vi "Binary to Nomal.vi"(0 "Module Type":T1=enum."NI 9215", 5 "Channel Calibration":cluster{"LSB Weight":u32, "Offset":i32}, 9 "Numeric":i32) -> (4 "Units":enum8{"mA", "V", "V/V", "Ohms"}(ring), 10 "data":dbl)   [LabVIEW 2018]
doc: "Converts a binary value to its nominal value equivalent.."
uses:
  <vilib>/LabVIEW Targets/FPGA/cRIO/shared/nicrio_ModuleControls/nicrio_calibrationModTypeEnum.ctl
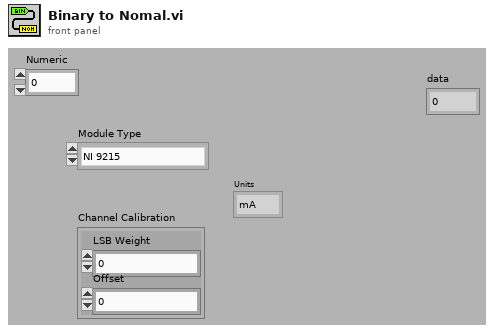
[diagram p1: front panel]
types:
  T1 = typedef "nicrio_calibrationModTypeEnum.ctl" = enum8{"NI 9201", "NI 9203 (4-20 mA range)", "NI 9203 (+/- 20 mA range)", "NI 9205", "NI 9206", "NI 9215", "NI 9221", "NI 9229", "NI 9233", "NI 9234", "NI 9237", "NI 9239", "NI 9263", "NI 9264", "NI 9265", "NI 9217", "NI 9236", "NI 9235", "NI 9225", "NI 9227", "NI 9269", "NI 9222", "NI 9223", "NI 9232", "NI 9381 (AI)", "NI 9381 (AO)", "NI 9220", "NI 9238", "NI 9218 (+/- 60 V range)", "NI 9218 (+/- 16 V range)", "NI 9218 (+/- 65 mV range)", "NI 9218 (+/- 5V IEPE range)", "NI 9218 (+/- 20 mA range)", "NI 9218 (+/- 22 mV/V range)", "NI 9260", "NI 9216", "NI 9226", "NI 9246", "NI 9247", "NI 9230", "NI 9266", "Ni 9775  (AI)", "NI 9775 (Trigger Level)", "NI 9775 (Hysteresis Level)", "NI 9684 (+/- 10 V range)", "NI 9684 (+/- 5 V range)"}
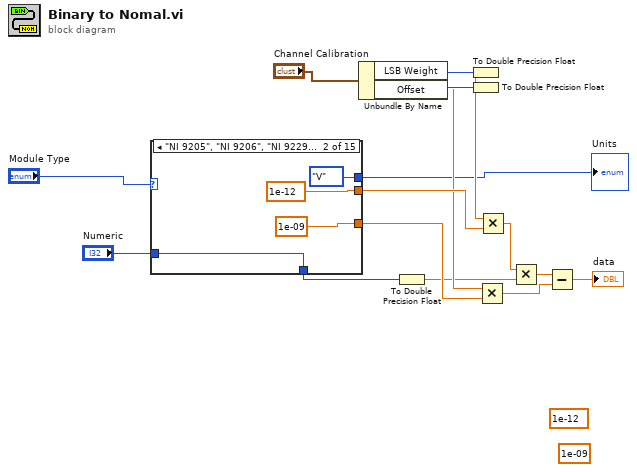
[diagram p0: block diagram]
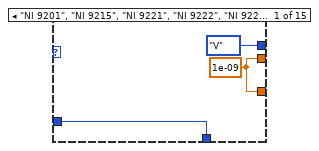
[diagram p2: hidden frame]
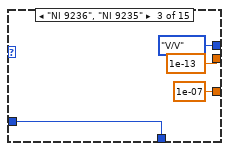
[diagram p3: hidden frame]
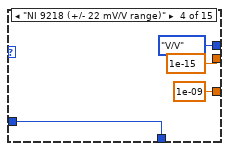
[diagram p4: hidden frame]
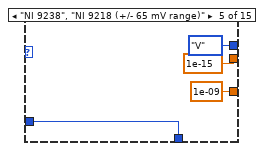
[diagram p5: hidden frame]
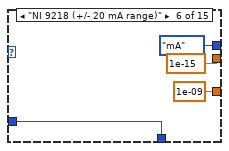
[diagram p6: hidden frame]
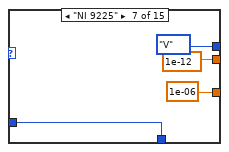
[diagram p7: hidden frame]
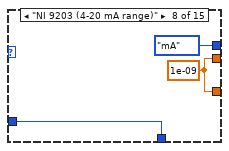
[diagram p8: hidden frame]
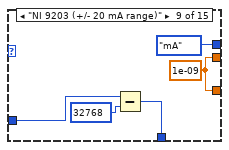
[diagram p9: hidden frame]
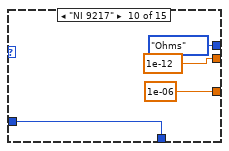
[diagram p10: hidden frame]
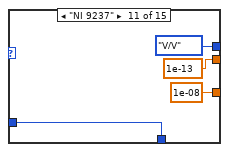
[diagram p11: hidden frame]
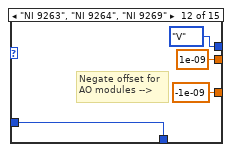
[diagram p12: hidden frame]
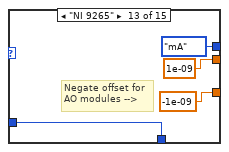
[diagram p13: hidden frame]
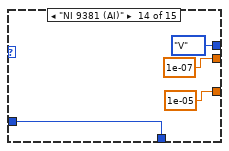
[diagram p14: hidden frame]
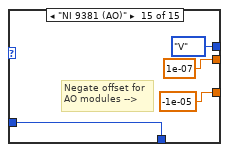
[diagram p15: hidden frame]
diagram:
  (unwired) 1e-09 ("y")
  (unwired) 1e-12 ("y")
  n1 = case shown="\"NI 9205\", \"NI 9206\", \"NI 9229\"..\"NI 9234\", \"NI 9239\", \"NI 9227\", \"NI 9232\", \"NI 9218 (+/- 60 V range)\", \"NI 9218 (+/- 16 V range)\", \"NI 9218 (+/- 5V IEPE range)\"" "Module Type" {
    tunnel: [w19 1e-12 ("y") 1e-13 ("y") 1e-15 ("y") 1e-15 ("y") 1e-15 ("y") 1e-12 ("y") w46 w50 1e-12 ("y") 1e-13 ("y") 1e-09 ("y") 1e-09 ("y") 1e-07 ("y") 1e-07 ("y")] -> w10
    tunnel: [w19 1e-09 ("y") 1e-07 ("y") 1e-09 ("y") 1e-09 ("y") 1e-09 ("y") 1e-06 ("y") w46 w50 1e-06 ("y") 1e-08 ("y") -1e-09 ("y") -1e-09 ("y") 1e-05 ("y") -1e-05 ("y")] -> w9
    tunnel: [enum8{"mA", "V"}."V" ("Units") enum8{"mA", "V"}."V" ("Units") enum8{"mA", "V", "V/V", "Ohms"}."V/V" ("Units") enum8{"mA", "V", "V/V", "Ohms"}."V/V" ("Units") enum8{"mA", "V", "V/V", "Ohms"}."V" ("Units") enum8{"mA", "V", "V/V", "Ohms"}."mA" ("Units") enum8{"mA", "V", "V/V", "Ohms"}."V" ("Units") enum8{"mA", "V"}."mA" ("Units") enum8{"mA", "V"}."mA" ("Units") enum8{"mA", "V", "V/V", "Ohms"}."Ohms" ("Units") enum8{"mA", "V", "V/V"}."V/V" ("Units") enum8{"mA", "V", "V/V"}."V" ("Units") enum8{"mA", "V", "V/V"}."mA" ("Units") enum8{"mA", "V", "V/V"}."V" ("Units") enum8{"mA", "V", "V/V"}."V" ("Units")] -> w5
    tunnel: "Numeric" -> [w17 w20 w26 w30 w34 w38 w40 w44 w49 w54 w56 w63 w64 w68 w72]
    tunnel: [w17 w20 w26 w30 w34 w38 w40 w44 w47 w54 w56 w63 w64 w68 w72] -> w4
    frame "NI 9201", "NI 9215", "NI 9221", "NI 9222", "NI 9223", "NI 9220", Default {
      w19 = 1e-09 ("y")
    }
    frame "NI 9205", "NI 9206", "NI 9229".."NI 9234", "NI 9239", "NI 9227", "NI 9232", "NI 9218 (+/- 60 V range)", "NI 9218 (+/- 16 V range)", "NI 9218 (+/- 5V IEPE range)" {
    }
    frame "NI 9236", "NI 9235" {
    }
    frame "NI 9218 (+/- 22 mV/V range)" {
    }
    frame "NI 9238", "NI 9218 (+/- 65 mV range)" {
    }
    frame "NI 9218 (+/- 20 mA range)" {
    }
    frame "NI 9225" {
    }
    frame "NI 9203 (4-20 mA range)" {
      w46 = 1e-09 ("y")
    }
    frame "NI 9203 (+/- 20 mA range)" {
      w50 = 1e-09 ("y")
      n2 = Subtract(x=w49, y=32768) -> (x-y=w47:i32)
    }
    frame "NI 9217" {
    }
    frame "NI 9237" {
    }
    frame "NI 9263", "NI 9264", "NI 9269" {
      # "Negate offset for AO modules -->"
    }
    frame "NI 9265" {
      # "Negate offset for AO modules -->"
    }
    frame "NI 9381 (AI)" {
    }
    frame "NI 9381 (AO)" {
      # "Negate offset for AO modules -->"
    }
  }
  "Units" <- w5
  n3 = Unbundle By Name("Channel Calibration") -> ("LSB Weight"=w15:u32, "Offset"=w13:i32)
  n4 = To Double Precision Float(number=w4) -> (double precision float=w6:dbl)
  n5 = To Double Precision Float(number=w15) -> (double precision float=w7:dbl)
  n6 = To Double Precision Float(number=w13) -> (double precision float=w8:dbl)
  n7 = Multiply(x=w8, y=w9) -> (x*y=w11:dbl)
  n8 = Multiply(x=w7, y=w10) -> (x*y=w14:dbl)
  n9 = Multiply(x=w14, y=w6) -> (x*y=w12:dbl)
  n10 = Subtract(x=w12, y=w11) -> (x-y=→"data":dbl)
